vi "9.vi"() -> ()   [LabVIEW 2023, in "2022.lvlib"]
uses:
  2022.lvlib
  <userlib>/_OpenG.lib/array/array.llb/Remove Duplicates from 1D Array (Variant)__ogtk.vi
panel:
  out "9_2 out array":cluster{"PosX":i32, "PosY":i32}[](array[cluster])
  out "9_2 result":i32
  out "9_1 result":i32
  out "9_1 out array":cluster{"PosX":i32, "PosY":i32}[](array[cluster])
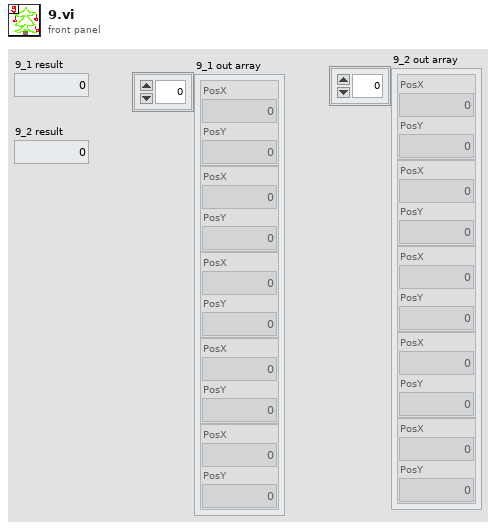
[diagram p1: front panel]
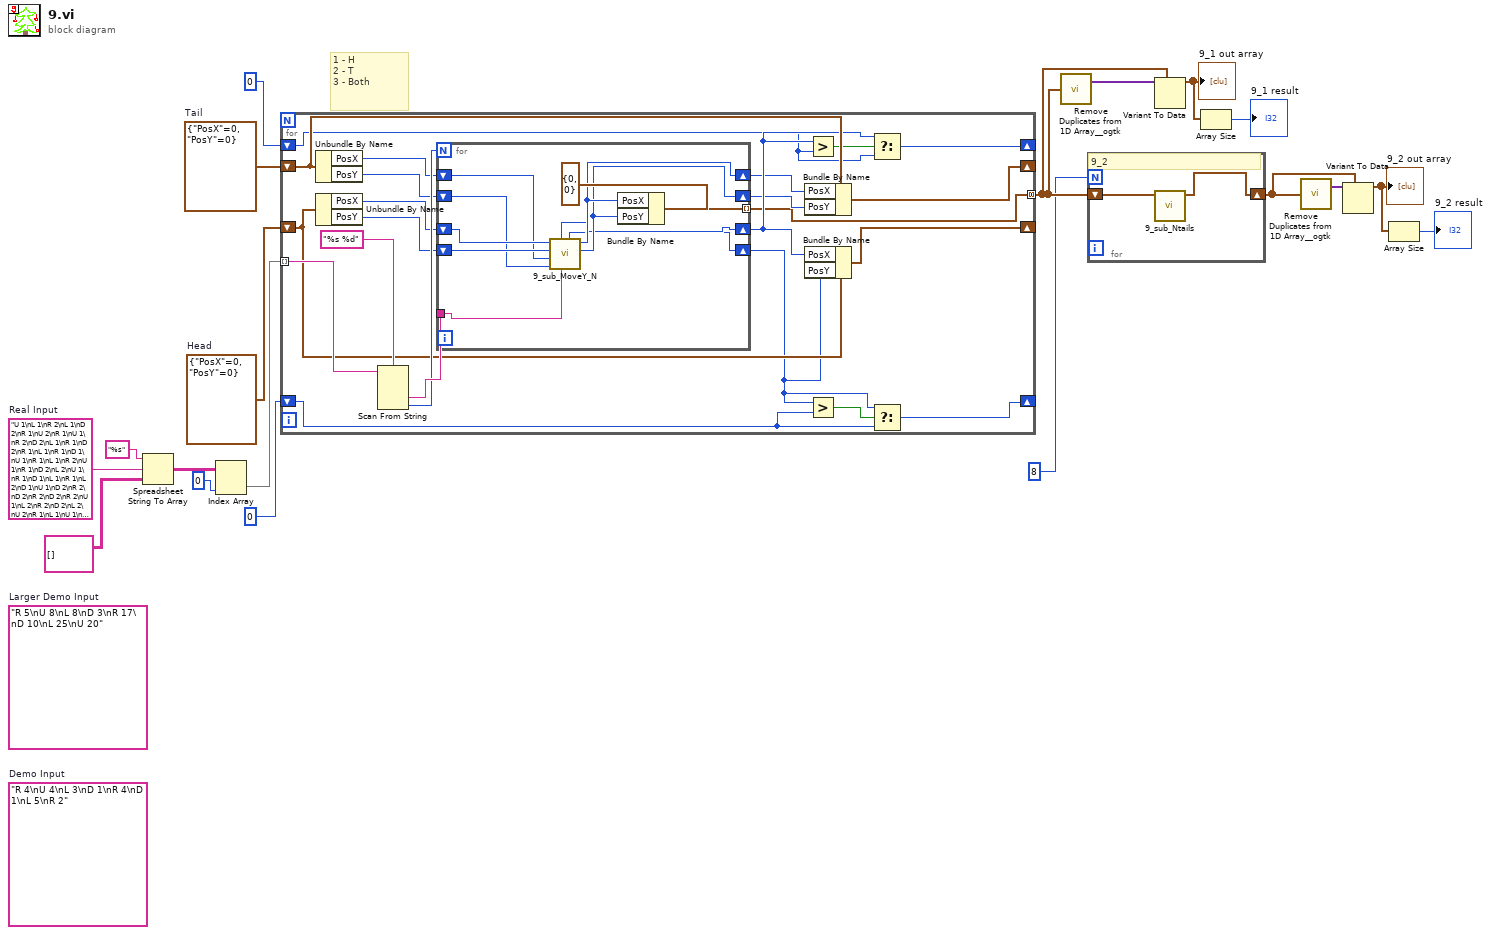
[diagram p0: block diagram]
diagram:
  (unwired) "R 5\nU 8\nL 8\nD 3\nR 17\nD 10\nL 25\nU 20"  # Larger Demo Input
  w13 = cluster{"PosX":i32, "PosY":i32} {"PosX"=0, "PosY"=0}  # Tail
  w14 = cluster{"PosX":i32, "PosY":i32} {"PosX"=0, "PosY"=0}  # Head
  (unwired) "R 4\nU 4\nL 3\nD 1\nR 4\nD 1\nL 5\nR 2"  # Demo Input
  w1 = "U 1\nL 1\nR 2\nL 1\nD 2\nR 1\nU 2\nR 1\nU 1\nR 2\nD 2\nL 1\nR 1\nD 2\nR 1\nL 1\nR 1\nD 1\nU 1\nR 1\nL 1\nR 2\nU 1\nR 1\nD 2\nL 2\nU 1\nR 1\nD 1\nL 1\nR 1\nL 2\nD 1\nU 1\nD 2\nR 2\nD 2\nR 2\nD 2\nR 2\nU 1\nL 2\nR 2\nD 2\nL 2\nU 2\nR 1\nL 1\nU 1\nR 1\nD 1\nR 1\nL 1\nR 1\nD 2\nL 2\nU 1\nR 1\nL 1\nR 1\nU 2\nD 2\nU 2\nL 1\nU 2\nL 1\nR 2\nU 2\nD 1\nL 1\nR 1\nL 2\nU 1\nD 2\nR 2\nU 2\nR 1\nL 1\nU 2\nR 2\nL 1\nR 2\nD 1\nU 2\nD 2\nR 2\nL 1\nR 1\nU 2\nD 2\nU 2\nD 1\nU 1\nR 2\nD 1\nR 1\nL 1\nD 2\nL 2\nU 2\nR 2\nU 1\nR 2\nU 1\nD 1\nR 2\nU 1\nR 1\nU 2\nR 2\nD 2\nL 2\nD 3\nR 2\nU 2\nR 2\nU 2\nL 3\nU 1\nL 1\nR 3\nD 2\nR 2\nU 1\nL 2\nD 2\nL 3\nU 3\nD 2\nR 3\nU 3\nR 2\nD 2\nU 3\nL 1\nU 2\nR 2\nL 1\nD 3\nU 1\nR 3\nL 2\nD 1\nU 2\nL 3\nR 3\nU 3\nL 1\nD 1\nR 3\nD 3\nR 1\nU 2\nR 3\nL 2\nR 1\nU 2\nL 3\nD 1\nR 3\nU 2\nD 2\nR 2\nD 3\nL 3\nD 1\nL 2\nD 1\nR 2\nL 1\nD 2\nU 1\nD 3\nU 1\nR 1\nU 1\nR 3\nL 3\nU 2\nD 3\nR 3\nU 1\nL 1\nR 1\nU 3\nL 2\nU 2\nD 3\nL 2\nD 1\nR 2\nD 2\nL 1\nR 2\nU 1\nD 3\nR 3\nD 2\nR 3\nL 3\nR 3\nD 1\nU 1\nR 1\nU 2\nD 2\nL 2\nD 3\nR 2\nD 3\nU 2\nL 2\nR 1\nU 3\nL 1\nD 1\nU 1\nD 2\nU 1\nL 3\nR 2\nD 1\nL 3\nU 1\nR 3\nD 2\nU 4\nD 1\nL 4\nR 2\nL 2\nR 2\nU 4\nR 1\nU 3\nL 2\nU 2\nR 3\nL 3\nD 3\nR 4\nD 4\nR 3\nD 1\nL 4\nD 4\nU 3\nD 3\nL 4\nR 4\nL 2\nR 3\nL 4\nD 3\nL 3\nU 1\nR 2\nU 1\nL 3\nU 4\nD 1\nL 2\nU 2\nL 1\nD 1\nR 2\nL 4\nR 3\nU 4\nR 1\nD 1\nR 1\nU 3\nD 4\nR 1\nU 4\nR 2\nD 2\nU 2\nR 2\nU 4\nL 1\nD 3\nL 4\nD 2\nL 2\nD 2\nU 4\nL 4\nR 1\nD 1\nR 3\nD 3\nL 4\nR 3\nD 2\nR 1\nD 1\nR 1\nU 1\nD 1\nL 1\nD 1\nR 2\nL 3\nD 1\nR 1\nL 4\nD 4\nR 4\nL 3\nD 4\nU 2\nL 1\nD 3\nU 2\nD 1\nR 2\nD 2\nL 2\nU 1\nD 4\nR 3\nU 4\nD 1\nR 3\nU 1\nD 1\nU 1\nR 1\nD 1\nR 3\nU 4\nR 4\nU 2\nL 1\nU 1\nL 3\nR 5\nD 2\nU 1\nR 3\nD 3\nR 1\nD 1\nL 5\nR 1\nD 1\nR 2\nU 3\nR 2\nL 4\nU 3\nD 4\nU 1\nR 3\nD 1\nR 2\nL 3\nR 3\nU 2\nL 5\nU 3\nR 4\nD 4\nR 2\nD 3\nR 2\nU 4\nL 5\nR 2\nL 3\nU 4\nL 5\nR 3\nD 3\nU 4\nR 2\nU 5\nR 2\nU 5\nD 1\nL 2\nD 2\nU 3\nR 3\nL 3\nU 3\nD 5\nR 4\nD 4\nL 4\nD 5\nR 1\nU 4\nL 2\nR 1\nD 3\nL 2\nR 2\nL 3\nR 2\nL 2\nD 3\nU 5\nD 5\nL 3\nR 5\nU 3\nL 3\nD 5\nL 4\nD 1\nL 2\nD 4\nU 4\nD 1\nR 1\nL 4\nR 3\nU 2\nL 3\nU 4\nD 4\nR 2\nD 4\nU 2\nD 4\nU 2\nL 4\nD 5\nL 4\nR 1\nL 2\nR 3\nD 2\nR 5\nL 1\nU 5\nR 1\nD 5\nL 1\nD 2\nU 5\nD 2\nU 1\nD 6\nU 2\nL 5\nD 2\nR 1\nD 1\nR 1\nD 5\nU 1\nD 5\nR 4\nL 3\nR 4\nU 1\nD 5\nU 5\nL 4\nU 5\nL 4\nU 5\nR 2\nL 6\nD 4\nL 1\nU 1\nR 6\nD 4\nL 1\nD 2\nR 2\nU 5\nR 5\nU 4\nL 5\nR 4\nD 4\nU 4\nD 1\nR 2\nL 5\nU 3\nR 1\nL 3\nU 6\nR 5\nL 2\nD 4\nR 4\nU 5\nR 2\nU 6\nL 4\nU 6\nR 2\nL 6\nD 5\nR 6\nU 1\nL 3\nU 4\nR 2\nL 5\nD 4\nL 6\nU 1\nD 1\nR 2\nD 5\nL 1\nR 5\nL 3\nU 5\nD 4\nU 5\nD 4\nU 2\nR 4\nL 3\nD 4\nL 5\nR 6\nU 6\nD 5\nU 2\nR 4\nD 5\nL 5\nR 3\nL 3\nD 3\nU 6\nL 1\nD 3\nR 2\nL 3\nR 2\nL 6\nD 1\nL 6\nD 4\nL 6\nR 4\nD 5\nL 3\nU 6\nR 5\nU 4\nD 1\nL 5\nU 1\nD 2\nU 2\nD 5\nR 7\nL 3\nU 5\nR 4\nL 5\nU 1\nR 2\nD 6\nL 6\nD 2\nL 1\nD 6\nU 2\nD 2\nU 2\nD 6\nL 1\nR 6\nU 7\nD 2\nL 3\nR 3\nU 6\nD 3\nR 4\nU 3\nL 7\nD 3\nU 6\nD 2\nU 1\nR 4\nL 1\nR 3\nU 5\nD 6\nR 2\nL 4\nD 5\nR 6\nL 5\nD 1\nR 3\nD 2\nL 7\nU 1\nR 5\nD 6\nU 6\nD 4\nU 6\nD 2\nL 2\nU 7\nD 1\nR 3\nU 3\nR 1\nL 6\nD 7\nL 4\nR 1\nD 7\nL 2\nU 6\nD 2\nR 6\nD 7\nU 7\nR 5\nL 1\nU 3\nR 5\nD 4\nU 2\nD 2\nL 6\nD 2\nU 7\nR 4\nL 7\nU 4\nD 6\nU 2\nD 6\nL 3\nU 5\nR 5\nD 4\nR 1\nD 6\nU 6\nR 3\nL 2\nU 1\nR 7\nD 4\nL 2\nD 4\nL 5\nU 3\nR 6\nL 3\nD 7\nR 7\nL 1\nU 4\nL 6\nR 7\nU 3\nR 1\nD 8\nL 3\nD 3\nU 3\nR 2\nL 6\nU 4\nL 2\nD 7\nL 5\nD 1\nR 3\nU 2\nL 6\nR 2\nU 1\nD 6\nU 4\nD 1\nU 8\nD 7\nR 3\nL 3\nR 1\nD 1\nR 5\nL 5\nR 6\nU 4\nR 4\nU 3\nR 4\nL 6\nR 4\nU 6\nL 5\nU 8\nL 1\nD 1\nL 4\nU 8\nR 2\nU 7\nL 4\nU 7\nL 7\nD 5\nU 1\nR 7\nU 7\nD 6\nR 5\nU 5\nD 2\nR 8\nL 1\nD 3\nL 5\nD 5\nR 1\nU 1\nR 4\nD 3\nR 1\nU 4\nR 8\nD 3\nL 4\nR 7\nL 4\nR 7\nL 7\nR 1\nL 1\nD 2\nL 6\nR 7\nD 5\nU 7\nL 8\nU 1\nL 8\nU 2\nR 6\nL 4\nU 1\nR 1\nU 3\nL 6\nD 7\nL 3\nD 2\nR 4\nU 5\nD 1\nU 2\nD 6\nL 6\nU 4\nD 1\nL 2\nR 4\nU 2\nL 1\nR 5\nL 3\nR 5\nU 7\nR 4\nL 4\nR 2\nD 4\nL 1\nR 2\nD 1\nL 2\nR 2\nU 2\nR 5\nL 7\nU 3\nR 1\nD 5\nU 7\nD 8\nR 7\nD 5\nU 2\nL 5\nD 4\nL 2\nD 8\nU 7\nD 3\nU 4\nL 9\nD 2\nU 7\nR 7\nD 9\nU 3\nR 2\nL 7\nU 5\nL 9\nD 5\nR 6\nD 5\nR 1\nD 1\nR 5\nD 3\nU 2\nR 5\nD 8\nU 4\nR 9\nU 5\nL 2\nU 2\nR 5\nD 9\nU 2\nD 3\nR 4\nD 5\nU 7\nL 2\nU 8\nR 7\nL 1\nU 4\nD 6\nR 8\nU 3\nD 4\nU 1\nR 5\nU 8\nD 9\nU 5\nD 9\nR 7\nD 3\nL 1\nD 4\nR 8\nD 8\nU 5\nD 7\nL 5\nU 1\nD 6\nL 7\nD 1\nR 1\nU 2\nL 3\nR 4\nL 1\nD 7\nL 3\nU 9\nR 1\nU 9\nL 7\nR 1\nU 5\nL 4\nU 8\nD 9\nU 3\nD 9\nR 5\nU 8\nL 9\nU 9\nD 7\nR 7\nL 2\nU 9\nR 7\nU 10\nD 7\nL 1\nD 2\nR 4\nD 9\nL 4\nD 7\nR 9\nU 1\nD 4\nU 8\nL 9\nR 9\nD 3\nR 2\nD 7\nU 2\nD 7\nU 1\nR 3\nD 1\nU 10\nD 5\nU 6\nD 1\nR 5\nD 6\nU 1\nR 6\nU 2\nD 5\nU 8\nL 9\nD 1\nU 9\nD 6\nL 10\nR 4\nD 1\nL 6\nR 1\nL 3\nD 4\nR 9\nD 7\nR 4\nD 8\nR 8\nL 5\nU 7\nR 3\nU 5\nD 4\nL 5\nD 7\nL 10\nU 3\nD 9\nR 7\nU 4\nD 3\nR 7\nU 5\nD 10\nR 1\nL 7\nU 7\nR 5\nU 4\nL 7\nD 6\nR 1\nD 1\nR 4\nL 3\nR 4\nD 3\nL 7\nD 7\nL 6\nR 4\nL 1\nD 2\nU 4\nD 8\nL 8\nR 1\nU 4\nD 1\nU 2\nL 1\nR 4\nU 7\nD 9\nU 4\nD 10\nU 5\nR 3\nD 6\nU 7\nD 6\nL 7\nR 7\nL 7\nR 6\nD 4\nU 4\nL 7\nU 9\nL 6\nD 2\nL 2\nU 10\nL 4\nU 3\nD 3\nL 5\nU 10\nD 10\nR 8\nD 2\nL 6\nD 9\nR 7\nL 8\nR 3\nU 1\nD 4\nU 2\nR 4\nU 5\nD 8\nU 6\nL 4\nU 9\nR 5\nU 8\nL 11\nD 11\nU 6\nD 4\nU 3\nR 7\nL 8\nR 5\nD 5\nU 5\nR 1\nU 10\nL 4\nD 6\nU 11\nR 3\nD 10\nU 10\nL 7\nR 11\nU 9\nL 10\nU 10\nL 11\nD 2\nL 9\nD 3\nL 11\nD 2\nU 1\nD 5\nL 6\nU 3\nD 10\nR 8\nU 10\nR 9\nL 1\nD 6\nU 6\nD 6\nL 8\nR 3\nU 1\nD 2\nL 6\nR 10\nU 7\nD 2\nL 5\nD 10\nU 5\nD 9\nR 4\nL 9\nD 6\nU 9\nR 5\nL 9\nU 1\nD 2\nR 2\nL 5\nR 4\nD 8\nU 8\nD 11\nL 4\nD 3\nU 1\nL 9\nR 8\nL 10\nR 8\nL 10\nU 10\nD 5\nR 11\nU 2\nR 8\nU 1\nL 6\nU 5\nD 2\nU 2\nR 3\nL 4\nR 1\nD 6\nL 6\nU 5\nR 1\nL 6\nD 1\nR 5\nL 2\nR 11\nD 5\nL 6\nR 1\nD 11\nU 9\nD 12\nU 8\nR 7\nL 6\nR 9\nU 7\nD 2\nR 5\nD 12\nL 10\nD 7\nL 5\nU 7\nD 9\nR 7\nU 8\nD 3\nU 8\nD 5\nU 1\nL 10\nU 7\nL 2\nR 5\nL 2\nU 1\nL 8\nR 2\nD 8\nR 9\nD 9\nR 11\nD 4\nR 3\nU 2\nD 9\nR 12\nU 11\nD 8\nR 6\nD 9\nU 3\nL 5\nR 1\nU 4\nR 4\nU 10\nR 11\nU 5\nR 9\nU 1\nR 5\nD 3\nR 8\nU 3\nR 6\nU 4\nR 3\nD 2\nL 2\nU 7\nL 2\nU 12\nD 10\nL 7\nU 6\nR 7\nU 1\nL 11\nU 12\nR 12\nL 12\nD 10\nR 9\nU 12\nL 6\nU 2\nL 7\nU 11\nR 7\nU 6\nL 3\nU 3\nD 1\nU 11\nR 1\nD 4\nR 10\nL 10\nR 6\nD 11\nR 1\nD 5\nL 1\nR 1\nL 4\nR 7\nU 12\nR 6\nL 10\nD 12\nL 4\nR 8\nU 5\nL 7\nR 10\nD 13\nU 7\nD 1\nR 1\nD 9\nR 3\nD 1\nL 4\nD 3\nR 5\nU 9\nR 11\nL 4\nR 1\nD 11\nL 2\nR 4\nD 7\nR 3\nU 2\nD 6\nR 2\nL 13\nR 5\nL 4\nR 4\nU 13\nR 3\nU 4\nR 3\nD 1\nL 3\nU 6\nL 8\nU 5\nR 4\nD 10\nL 3\nU 10\nR 11\nD 11\nU 2\nD 2\nR 4\nU 2\nD 1\nR 10\nU 5\nL 9\nU 11\nR 10\nD 4\nL 1\nU 5\nR 4\nU 6\nR 9\nD 12\nL 10\nR 5\nL 5\nD 9\nU 2\nR 7\nU 2\nR 5\nL 8\nD 5\nR 1\nD 5\nR 8\nU 11\nR 7\nL 13\nU 10\nD 3\nU 1\nD 2\nL 1\nD 12\nL 9\nD 12\nR 5\nU 8\nR 6\nL 6\nR 5\nU 7\nL 10\nD 5\nU 11\nD 4\nU 8\nR 7\nU 8\nR 2\nL 10\nD 5\nL 10\nD 3\nU 13\nD 11\nU 3\nR 10\nU 9\nD 7\nU 6\nR 1\nU 9\nR 11\nD 7\nR 6\nU 9\nR 6\nU 12\nD 6\nR 13\nL 14\nU 10\nR 9\nL 13\nR 7\nD 9\nU 12\nL 8\nD 5\nR 3\nU 5\nR 10\nL 4\nD 5\nR 4\nD 2\nL 12\nR 8\nD 9\nR 5\nD 7\nU 5\nD 11\nL 13\nD 12\nR 2\nU 5\nL 1\nU 2\nL 6\nU 9\nD 10\nL 3\nD 8\nR 12\nU 9\nR 9\nU 9\nR 8\nU 6\nL 10\nU 5\nR 9\nD 2\nU 12\nD 3\nR 12\nL 10\nD 5\nL 7\nD 9\nL 5\nR 7\nD 8\nU 10\nL 11\nR 9\nL 13\nR 8\nU 9\nD 8\nU 9\nR 10\nL 4\nU 1\nD 10\nL 1\nD 4\nL 1\nU 13\nR 8\nL 3\nD 5\nR 5\nU 4\nR 5\nU 6\nL 14\nR 5\nU 8\nL 7\nD 7\nR 4\nU 4\nL 14\nU 7\nR 14\nD 3\nU 10\nL 7\nR 5\nL 5\nR 15\nL 3\nD 15\nL 6\nR 3\nL 10\nU 7\nL 2\nR 7\nL 1\nR 8\nU 12\nD 6\nU 11\nD 12\nU 9\nR 2\nD 14\nL 4\nU 9\nD 15\nR 8\nD 9\nL 9\nD 14\nU 5\nR 14\nD 15\nR 6\nL 3\nU 13\nR 13\nU 5\nD 14\nL 2\nD 12\nU 6\nR 5\nU 5\nL 6\nR 5\nD 12\nU 9\nL 7\nD 15\nR 5\nU 7\nD 1\nR 2\nL 11\nU 8\nR 3\nD 3\nU 6\nD 15\nU 2\nD 11\nR 6\nU 9\nD 7\nU 3\nL 13\nU 3\nL 15\nR 10\nL 6\nD 15\nL 3\nU 5\nR 13\nD 13\nL 5\nR 8\nD 2\nR 8\nL 9\nR 7\nL 5\nU 3\nD 11\nR 13\nU 15\nD 5\nR 4\nU 11\nR 14\nL 1\nU 6\nL 13\nR 14\nL 12\nD 5\nR 3\nD 4\nR 5\nU 8\nR 11\nD 8\nU 5\nR 9\nD 8\nR 4\nU 5\nL 7\nD 6\nU 4\nL 2\nD 15\nU 5\nR 16\nL 4\nR 1\nD 12\nL 2\nR 6\nD 6\nR 14\nU 6\nL 14\nR 12\nD 8\nR 1\nU 2\nR 3\nD 7\nR 4\nL 2\nU 6\nL 1\nU 7\nL 12\nR 11\nD 13\nU 16\nR 15\nD 14\nU 13\nD 15\nR 11\nU 12\nR 5\nD 8\nR 2\nL 14\nR 10\nL 16\nU 10\nD 13\nL 11\nU 10\nR 5\nD 7\nL 15\nD 12\nL 4\nR 16\nU 8\nR 8\nL 7\nU 9\nR 7\nU 16\nR 2\nU 5\nR 5\nD 4\nL 7\nD 5\nL 4\nU 13\nD 9\nR 2\nD 2\nU 5\nL 3\nD 16\nR 13\nL 10\nR 7\nL 9\nR 3\nL 5\nD 10\nL 10\nR 2\nL 13\nR 5\nL 11\nR 16\nU 12\nR 11\nD 12\nR 7\nL 2\nU 12\nD 11\nU 12\nL 1\nR 6\nU 3\nL 3\nD 1\nR 5\nU 6\nL 15\nR 8\nD 5\nL 16\nD 13\nR 15\nD 14\nR 4\nU 15\nR 5\nL 8\nD 12\nU 11\nD 13\nL 9\nD 13\nL 7\nU 9\nR 15\nU 13\nD 16\nR 6\nL 8\nR 7\nU 4\nR 10\nU 7\nD 10\nU 8\nD 7\nL 17\nR 7\nL 8\nD 5\nL 5\nU 15\nD 6\nL 1\nD 2\nR 17\nL 6\nD 15\nR 4\nL 2\nR 10\nD 4\nR 6\nD 11\nU 1\nL 17\nD 11\nU 6\nD 17\nR 15\nL 13\nD 9\nR 12\nU 13\nR 2\nL 12\nD 1\nR 17\nU 13\nD 15\nU 7\nR 8\nD 6\nR 8\nD 16\nU 16\nD 2\nU 1\nR 7\nU 15\nL 7\nR 12\nU 10\nD 4\nR 17\nD 11\nR 12\nD 8\nL 3\nR 3\nD 5\nR 17\nL 15\nU 11\nR 1\nL 4\nR 6\nD 6\nU 2\nL 1\nD 2\nU 1\nD 11\nL 1\nR 11\nD 7\nU 16\nL 14\nU 5\nR 13\nD 9\nU 17\nD 3\nR 12\nU 16\nR 10\nL 17\nD 5\nU 16\nD 12\nL 2\nR 16\nL 17\nU 4\nR 15\nD 4\nL 11\nU 3\nR 17\nD 8\nR 7\nD 15\nR 14\nD 6\nR 5\nL 1\nD 5\nL 11\nD 5\nU 13\nL 13\nU 8\nD 8\nL 13\nD 1\nL 10\nU 14\nR 7\nL 11\nD 4\nR 16\nD 3\nL 9\nR 3\nD 4\nL 4\nU 2\nR 13\nD 18\nU 15\nD 7\nL 18\nU 3\nD 17\nU 13\nR 9\nL 8\nR 9\nU 16\nR 14\nD 17\nL 16\nR 3\nU 4\nD 1\nR 8\nD 14\nL 14\nU 17\nL 16\nR 15\nD 9\nU 13\nR 14\nU 9\nD 13\nR 2\nL 3\nD 8\nU 5\nR 1\nL 5\nR 4\nU 8\nL 7\nU 5\nR 11\nD 17\nL 4\nU 3\nR 1\nU 18\nD 1\nU 6\nR 2\nD 16\nU 15\nD 8\nL 13\nR 2\nU 16\nL 9\nD 1\nU 9\nR 5\nL 16\nD 2\nL 2\nR 8\nD 17\nR 13\nU 5\nR 6\nU 2\nL 12\nR 2\nD 14\nR 14\nL 11\nR 1\nL 9\nD 18\nL 4\nU 4\nD 15\nL 14\nR 15\nU 6\nD 3\nR 15\nL 12\nU 3\nD 12\nU 13\nL 6\nU 17\nD 6\nL 10\nR 16\nL 7\nU 2\nD 1\nR 10\nU 11\nR 1\nU 19\nD 5\nL 11\nD 14\nL 17\nU 16\nL 13\nR 4\nL 16\nD 10\nL 4\nD 9\nR 19\nL 19\nR 12\nL 12\nD 8\nL 6\nD 14\nU 7\nD 13\nU 18\nD 13\nU 6\nD 6\nR 18\nU 18\nD 15\nL 14\nR 7\nD 11\nR 4\nL 14\nR 5\nD 4\nL 12\nD 16\nR 17\nU 15\nL 9\nU 10\nR 7\nD 10\nL 3\nU 15\nL 1\nD 15\nU 1\nD 12\nL 4\nD 10\nU 6\nR 6\nL 11\nD 5\nR 1\nD 11\nU 16\nL 16\nR 19\nU 8\nR 11\nD 17\nL 19\nR 6\nU 7\nR 2\nD 9\nR 11\nD 17\nU 17\nD 4\nR 8\nD 6\nU 10\nR 3\nL 17\nD 5\nR 19\nU 1\nL 5\nU 5\nD 6\nU 6\nL 18\nR 18\nL 4\nR 12\nD 14\nL 17\nR 8\nL 13\nR 6\nL 14\nD 3\nR 13\nL 16\nD 14\nU 6\nD 6"  # Real Input
  # "1 - H\n2 - T\n3 - Both"
  n1 = Spreadsheet String To Array(format string="%s", spreadsheet string=w1, array type (2D Dbl)=string[][] []) -> (array=w17:string[][])  [unwired: 1 in]
  n2 = Index Array(array=w17, index (col)=0 ("disabled index (col)")) -> (element=w15:string[])  [unwired: 1 in]
  n3 = for {
    tunnel: w15 -> [w42] mode=indexing
    shift-right: [w35] -> _
    shift-left: w14 -> [w38]
    shift-right: [w31] -> _
    shift-left: w13 -> [w34]
    shift-right: [w27] -> _
    shift-left: 0 ("PosX") -> [w28]
    shift-right: [w23] -> _
    shift-left: 0 ("PosY") -> [w24]
    tunnel: [w20] -> w7 mode=concatenating
    n4 = Unbundle By Name(w34) -> ("PosX"=w33:i32, "PosY"=w32:i32)
    n5 = Unbundle By Name(w38) -> ("PosX"=w37:i32, "PosY"=w36:i32)
    n6 = Scan From String(format string="%s %d", input string=w42) -> (output 1=w40:string, output 2=w39:i32)  [unwired: 4 in, 3 out]
    n7 = for {
      N: w39 -> [_]
      shift-right: [w44] -> w29
      shift-left: w37 -> [w53]
      shift-right: [w43] -> w25
      shift-left: w36 -> [w52]
      shift-right: [w48] -> w22
      shift-left: w33 -> [w51]
      shift-right: [w47] -> w21
      shift-left: w32 -> [w50]
      tunnel: w40 -> [w45]
      tunnel: [w46] -> w20 mode=indexing
      n8 = call "9_sub_MoveY_N.vi"("Dir"=w45, "T_y"=w50, "T_x"=w51, "H_y"=w52, "H_x"=w53) -> ("T_y 2"=w47:i32, "T_x 2"=w48:i32, "H_y 2"=w43:i32, "H_x 2"=w44:i32)  [unwired: 3 in]
      n9 = Bundle By Name(cluster=cluster{"PosX":i32, "PosY":i32} {"PosX"=0, "PosY"=0} ("Tail"), "PosX"=w48, "PosY"=w47) -> (w46:cluster{"PosX":i32, "PosY":i32})
    }
    n10 = Bundle By Name(cluster=w34, "PosX"=w22, "PosY"=w21) -> (w31:cluster{"PosX":i32, "PosY":i32})
    n11 = Bundle By Name(cluster=w38, "PosX"=w29, "PosY"=w25) -> (w35:cluster{"PosX":i32, "PosY":i32})
    n12 = Greater?(x=w29, y=w28) -> (0:w30:bool)
    n13 = Greater?(x=w25, y=w24) -> (0:w26:bool)
    n14 = Select(t=w29, s=w30, f=w28) -> (s? t:f=w27:i32)
    n15 = Select(t=w25, s=w26, f=w24) -> (s? t:f=w23:i32)
  }
  n16 = call-poly <userlib>:"Remove Duplicates from 1D Array__ogtk.vi"("Input Array"=w7) -> ("Output Array"=w10:variant[])  [unwired: 1 out]
  n17 = for {
    N: 8 -> [_]
    shift-right: [w54] -> w2
    shift-left: w7 -> [w55]
    # "9_2"
    n18 = call "9_sub_Ntails.vi"("Array"=w55) -> ("Array 2"=w54:cluster{"PosX":i32, "PosY":i32}[])  [unwired: 10 in]
  }
  n19 = Variant To Data(type=w7, Variant=w10) -> (data=w9:cluster{"PosX":i32, "PosY":i32}[])  [unwired: 1 in, 1 out]
  "9_1 out array" <- w9
  n20 = Array Size(array=w9) -> (size(s)=→"9_1 result":i32)
  n21 = call-poly <userlib>:"Remove Duplicates from 1D Array__ogtk.vi"("Input Array"=w2) -> ("Output Array"=w3:variant[])  [unwired: 1 out]
  n22 = Variant To Data(type=w2, Variant=w3) -> (data=w4:cluster{"PosX":i32, "PosY":i32}[])  [unwired: 1 in, 1 out]
  "9_2 out array" <- w4
  n23 = Array Size(array=w4) -> (size(s)=→"9_2 result":i32)
